vi "CalibrationAndMeasureTest.vi"() -> ()   [LabVIEW 2019]
panel:
  out "Image 3":T1(plugin-control)
  out "Circles Data (calibrated) (Circle Detection 1)":T2(array[cluster])
  out "Image":T1(plugin-control)
  in  "Stop Button":bool
  out "Image 2":T1(plugin-control)
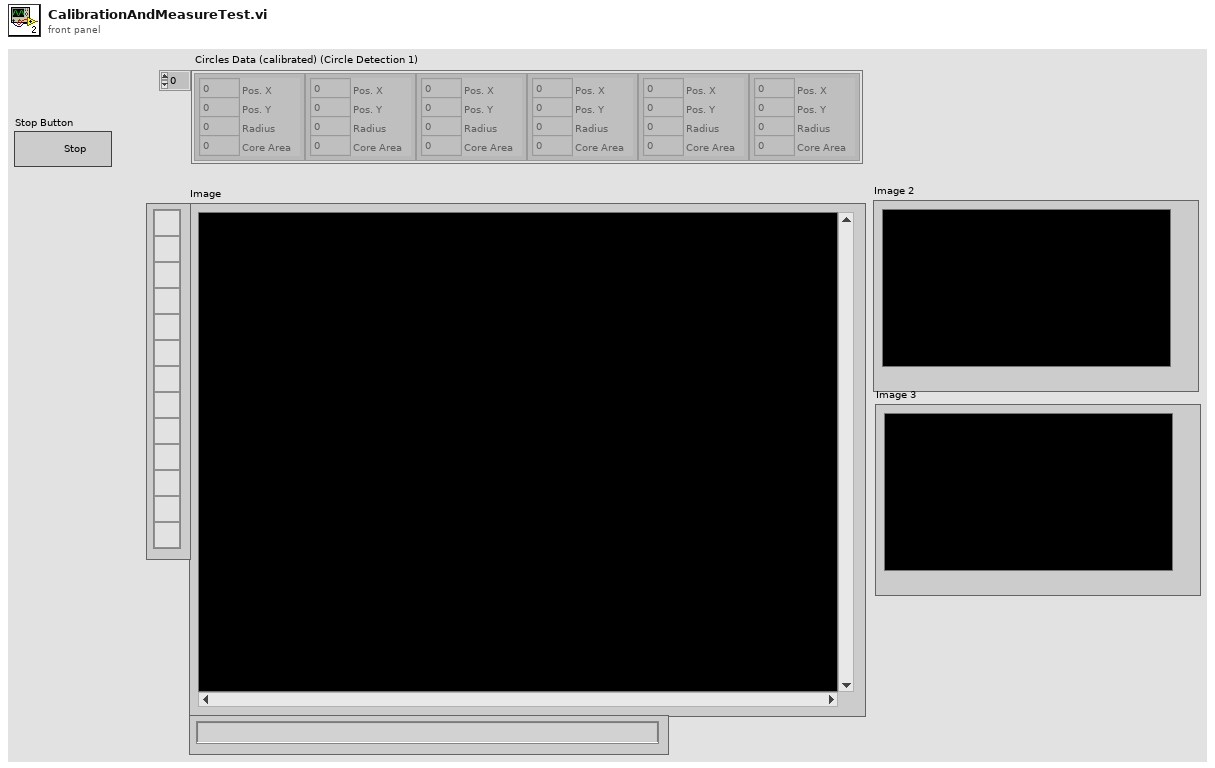
[diagram p1: front panel]
types:
  T1 = typedef "IMAQ Image.ctl" = refnum<image>
  T2 = cluster{"Pos. X":i32, "Pos. Y":i32, "Radius":i32, "Core Area":i32}[]
  T3 = typedef "Image Type" = u32
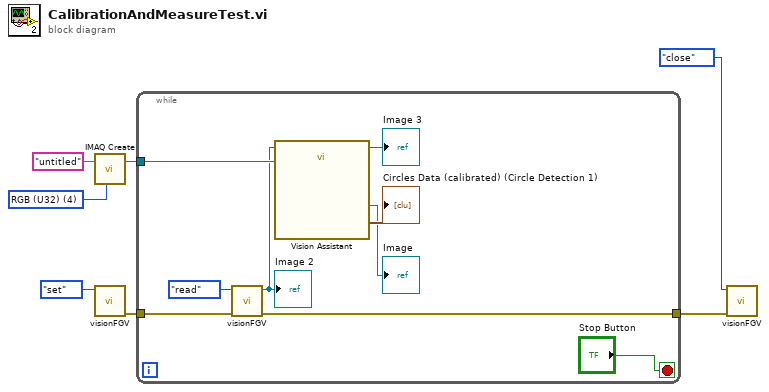
[diagram p0: block diagram]
diagram:
  w1 = T3 4 items=["Grayscale (U8)", "Grayscale (I16)", "Grayscale (SGL)", "Complex (CSG)", "RGB (U32)", "HSL (U32)", "RGB (U64)", "Grayscale (U16)"] ("Image Type")
  n1 = call "IMAQ Create"("Image Name"="untitled", "Image Type"=w1) -> ("New Image"=w2:T1)  [unwired: 3 in, 1 out]
  n2 = call "visionFGV.vi"("Function"=enum16{"set", "read", "close"}."set") -> ("error out"=w5:errorcluster)  [unwired: 9 in, 1 out]
  n3 = while {
    tunnel: w5 -> [w15]
    tunnel: [w14] -> w4
    tunnel: w2 -> [w13]
    stop <- "Stop Button" stop-if-true
    n4 = call "visionFGV.vi"("Error In"=w15, "Function"=enum16{"set", "read", "close"}."read") -> ("error out"=w14:errorcluster, "Image Out fgv"=w11:T1)  [unwired: 8 in]
    "Image 2" <- w11
    n5 = call "Vision Assistant"("Image In"=w11, "Image Dst"=w13) -> ("Image Out"=→"Image 3":T1, "Circles Data (calibrated) (Circle Detection 1)"=→"Circles Data (calibrated) (Circle Detection 1)":T2, "Image Buffer (Image Buffer 2)"=→"Image":T1)  [unwired: 22 in, 1 out]
  }
  n6 = call "visionFGV.vi"("Error In"=w4, "Function"=enum16{"set", "read", "close"}."close") -> ()  [unwired: 8 in, 2 out]
